vi "Instrument input.vi"(0 "Command":string, 11 "Error in":errorcluster) -> (4 "Response":string, 15 "Error out":errorcluster)   [LabVIEW 2020]
doc: "This VI gets in commands from user as SOURce and MEASure and the calls a subVI to write and get the values from the file to return and also logs this event with time"
panel:
  # "This VI give commands from user to another VI to store the data and then \nretrives it based on the command input"
  # "Command Input:\n1. Write:  SOURce:VOLTage/CURRent:DC ?\n2. Read:   MEASure:VOLTage/CURRent:DC"
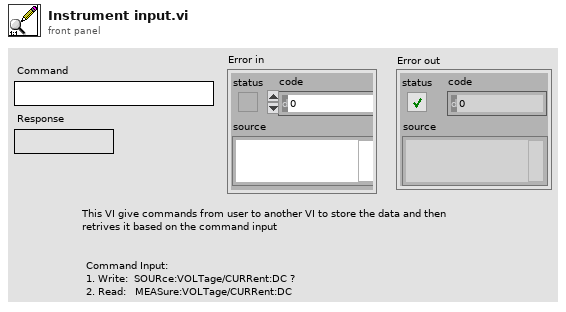
[diagram p1: front panel]
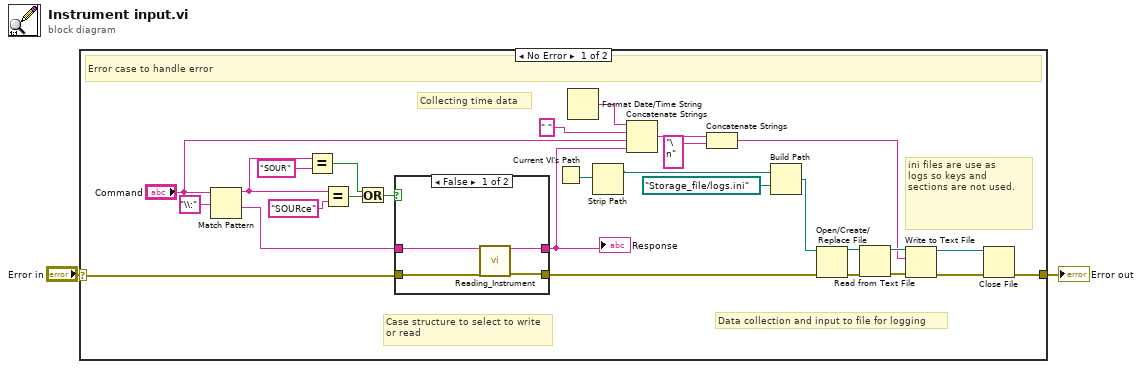
[diagram p0: block diagram]
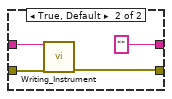
[diagram p2: hidden frame]
diagram:
  n1 = case shown="No Error" "Error in" {
    selector: "Error in" -> [w11 w39]
    tunnel: [w21 w39] -> w2
    frame No Error {
      # "Collecting time data"
      # "ini files are use as\nlogs so keys and \nsections are not used."
      # "Case structure to select to write\nor read"
      # "Data collection and input to file for logging"
      # "Error case to handle error"
      n2 = Match Pattern(string="Command", regular expression="\\:") -> (before substring=w7:string, after substring=w29:string)  [unwired: 1 in, 2 out]
      n3 = Equal?(x=w7, y="SOUR") -> (x = y?=w3:bool)
      n4 = Equal?(x=w7, y="SOURce") -> (x = y?=w4:bool)
      n5 = Or(x=w3, y=w4) -> (x .or. y?=w5:bool)
      n6 = case shown="False" w5 {
        tunnel: w29 -> [w34 w35]
        tunnel: [w33 "" ("String 3")] -> w22
        tunnel: [w31 w36] -> w12
        tunnel: w11 -> [w32 w37]
        frame False {
          n7 = call "Reading_Instrument.vi"("Read String"=w34, "error in"=w32) -> ("Readed Data"=w33:string, "error out"=w31:errorcluster)  [unwired: 12 in]
        }
        frame True, Default {
          n8 = call "Writing_Instrument.vi"("Write String"=w35, "error in"=w37) -> ("error out"=w36:errorcluster)  [unwired: 13 in]
        }
      }
      "Response" <- w22
      n9 = Current VI's Path() -> (path=w26:path)
      n10 = Format Date/Time String() -> (date/time string=w10:string)  [unwired: 3 in]
      n11 = Strip Path(path=w26) -> (stripped path=w20:path)  [unwired: 1 out]
      n12 = Concatenate Strings(w10, " " ("string"), "Command", w22) -> (w15:string)
      n13 = Concatenate Strings(w15, "\n" ("string")) -> (w13:string)
      n14 = Build Path(base path=w20, name or relative path=path "Storage_file/logs.ini") -> (appended path=w24:path)
      n15 = Open/Create/Replace File(file path (use dialog)=w24, error in=w12) -> (refnum out=w17:refnum<file>, error out=w19:errorcluster)  [unwired: 4 in, 1 out]
      n16 = Read from Text File(file (use dialog)=w17, error in=w19) -> (refnum out=w16:refnum<file>, error out=w18:errorcluster)  [unwired: 2 in, 2 out]
      n17 = Write to Text File(file (use dialog)=w16, text=w13, error in=w18) -> (refnum out=w27:refnum<file>, error out=w28:errorcluster)  [unwired: 1 in, 1 out]
      n18 = Close File(refnum=w27, error in=w28) -> (error out=w21:errorcluster)  [unwired: 1 out]
    }
    frame Error {
    }
  }
  "Error out" <- w2
